vi "Write Steps State.vi"(8 "error in (no error)":errorcluster, 10 "Steps State":T1[](array[typedef]), 11 "Parallel Step in":refnum<class "Parallel Step.lvclass">) -> (0 "error out":errorcluster, 3 "Parallel Step out":refnum<class "Parallel Step.lvclass">)   [LabVIEW 2015, in "Parallel Step.lvclass"]
uses:
  Parallel Step.lvclass
  Step/StepState.ctl
  Step/Step State Enum.ctl
  Parallel Step.lvclass/Parallel Step.ctl
  Step/Step.lvclass
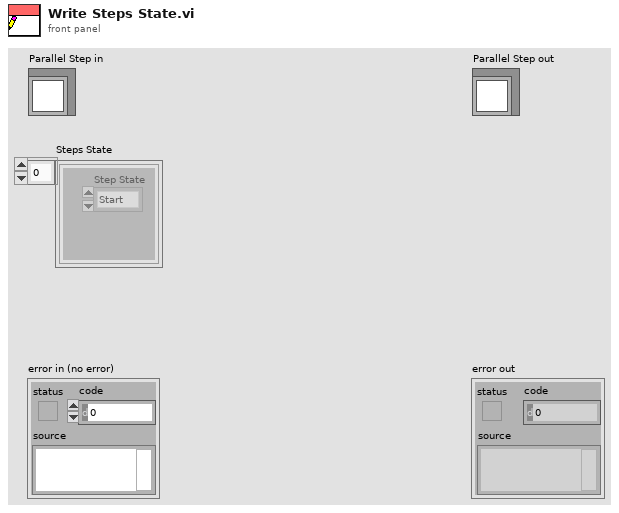
[diagram p1: front panel]
types:
  T1 = typedef "Step.lvclass/StepState.ctl" = cluster{"Step State":T2}
  T2 = typedef "Step.lvclass/Step State Enum.ctl" = enum16{"Start", "Skipped", "Completed", "Running", "Aborted"}
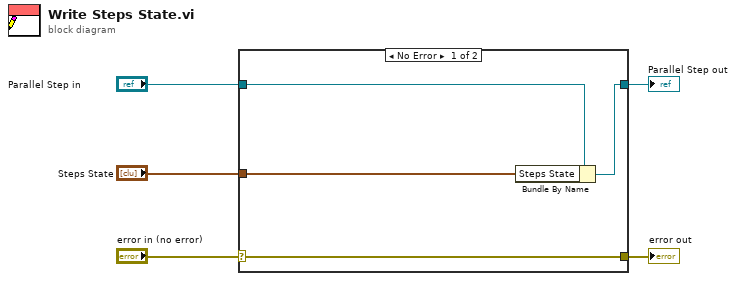
[diagram p0: block diagram]
diagram:
  n1 = case shown="No Error" "error in (no error)" {
    selector: "error in (no error)" -> [w9 w10]
    tunnel: [w9 w10] -> w4
    tunnel: [w7 w11] -> w2
    tunnel: "Parallel Step in" -> [w8 w11]
    tunnel: "Steps State" -> [w6 _]
    frame No Error {
      n2 = Bundle By Name(cluster=w8, "Steps State"=w6) -> (w7:refnum<class "Parallel Step.lvclass">)
    }
    frame Error {
    }
  }
  "error out" <- w4
  "Parallel Step out" <- w2
